vi "Tilted Logistic Square Pulse Fit Result File String.vi"(8 "error in (no error)":errorcluster, 9 "Delta Best Fit Parameters":dbl[](array[numeric]), 10 "Fit Output":T1={"best nonlinear fit"=[], "best fit parameters"=[], "R^2"=0.0, "RMSE"=0.0, "error out"={"status"=FALSE, "code"=0, "source"=""}, "Fitting Method"=enum."Least Square", "number of function calls"=0, "number of iterations"=0, "covariance"=[], "Chi 2"=0.0, "DOF"=0, "Fit Convergence Criterion"=enum."Continue", "Fitting Algorithm"=enum."Levenberg-Marquardt", "Weighted Fit"=enum."Unweighted", "Gradient"=0.0, "|Delta Chi 2|"=0.0, "|Delta Chi 2|/Chi 2"=0.0, "Max |Delta a| /|a|"=0.0, "Lambda"=-1.0, "RSS"=0.0, "AIC"=0.0, "BIC"=0.0, "Max number of function calls"=0, "Max number of iterations"=0, "IRF"={"X Array"=[], "Y Array"=[]}, "IRF Normalization Factor"=0.0, "Decay Normalization Factor"=0.0, "Number of offset fits"=0, "Weighted Chi2"=-1.0, "Unweighted Chi2"=-1.0}, 11 "ROI Descriptor":T8 {"Contours"."Type" items=["No Selection", "Point", "Line", "Rectangle", "Oval", "Polygon", "Freehand Region", "Annulus", "Unused2", "Unused3", "Broken Line", "Freehand Line", "Rotated Rectangle"]}) -> (0 "error out":errorcluster, 3 "Result String":string, 5 "Header String":string="ROI_x\tROI_y\tAL\tAL_err\tAU\tAU_err\tx0R\tx0R_err\tdxR\tdxR_err\tx0F\tx0F_err\tdxF\tdxF_err\tR^2\tRMSE\tMethod\tCalls\tIterations")   [LabVIEW 2021, in "Fits.lvlib"]
doc: "Creates Notebook output for a tilted logistic square gate fit."
uses:
  Fits.lvlib
  Non-linear Fit Output v4.ctl
  Nonlinear Fit Method.ctl
  <vilib>/Analysis/Matrix/Datatypes/RealMatrix.ctl
  Convergence Criteria.ctl
  Non-linear Fitting Algorithm.ctl
  IRF(X)PSED/Fit Weights Type v2.ctl
  Graphs/XY Graph/XY Graph Plot Data.ctl
  <vilib>/Analysis/Matrix/NI_Matrix.lvlib
  Graphs/XY Graph/XY Graph Add-Ons.lvlib
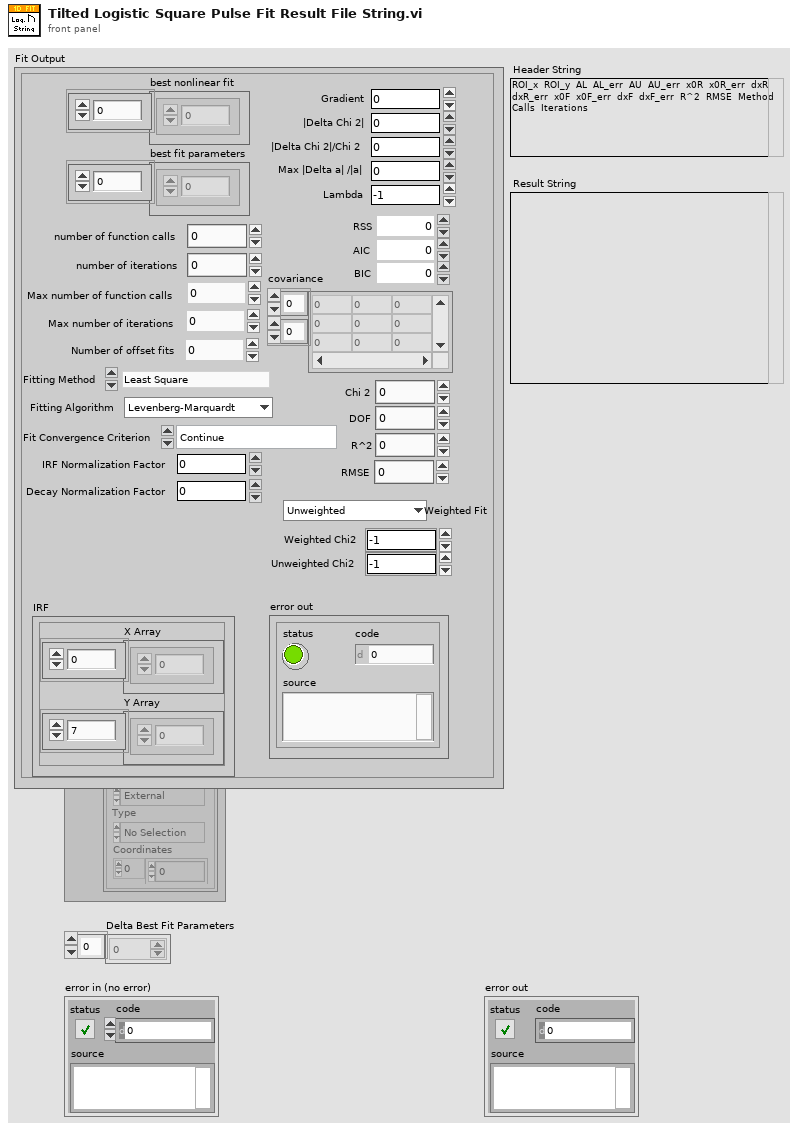
[diagram p1: front panel]
types:
  T1 = typedef "Fits.lvlib/Non-linear Fit Output v4.ctl" = cluster{"best nonlinear fit":dbl[], "best fit parameters":dbl[], "R^2":dbl, "RMSE":dbl, "error out":errorcluster, "Fitting Method":T2, "number of function calls":i32, "number of iterations":i32, "covariance":T3, "Chi 2":dbl, "DOF":i32, "Fit Convergence Criterion":T4, "Fitting Algorithm":T5, "Weighted Fit":T6, "Gradient":dbl, "|Delta Chi 2|":dbl, "|Delta Chi 2|/Chi 2":dbl, "Max |Delta a| /|a|":dbl, "Lambda":dbl, "RSS":dbl, "AIC":dbl, "BIC":dbl, "Max number of function calls":i32, "Max number of iterations":i32, "IRF":T7, "IRF Normalization Factor":dbl, "Decay Normalization Factor":dbl, "Number of offset fits":i32, "Weighted Chi2":dbl, "Unweighted Chi2":dbl}
  T2 = typedef "Fits.lvlib/Nonlinear Fit Method.ctl" = enum16{"Least Square", "Least Absolute Residual", "Bisquare", "MLE"}
  T3 = typedef "NI_Matrix.lvlib/RealMatrix.ctl" = dbl[][]
  T4 = typedef "Fits.lvlib/Convergence Criteria.ctl" = enum16{"Continue", "Tolerances Exceeded", "Max Time Exceeded", "Max Iterations Exceeded", "Max Function Evaluations Exceeded", "Scale Range Exceeded"}
  T5 = typedef "Fits.lvlib/Non-linear Fitting Algorithm.ctl" = enum16{"Levenberg-Marquardt", "Trust-Region Dogleg"}
  T6 = typedef "Fits.lvlib/Fit Weights Type v2.ctl" = enum16{"Unweighted", "1/Variance (Neyman)", "1/Variance (Pearson)", "Best of All"}
  T7 = typedef "XY Graph Add-Ons.lvlib/XY Graph Plot Data.ctl" = cluster{"X Array":dbl[], "Y Array":dbl[]}
  T8 = typedef "ROI Descriptor" = cluster{"Global Rectangle":i32[], "Contours":cluster{"ID":enum32{"External", "Internal"}, "Type":u32, "Coordinates":i32[]}[]}
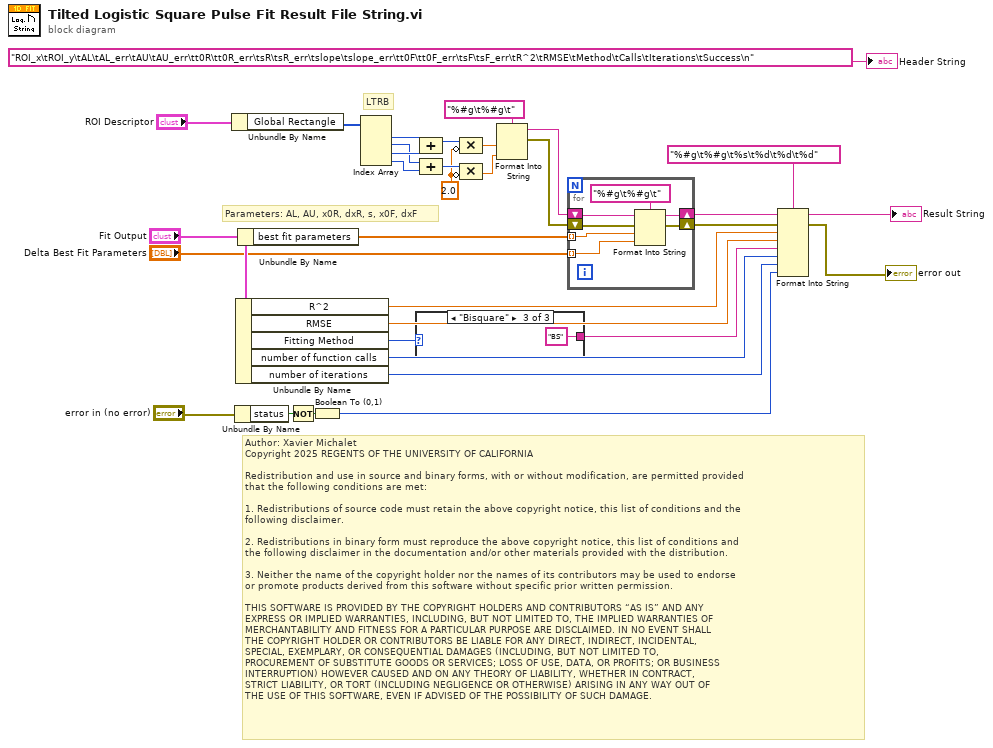
[diagram p0: block diagram]
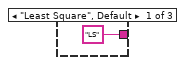
[diagram p2: hidden frame]
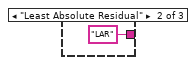
[diagram p3: hidden frame]
diagram:
  w7 = 2.0 ("value")
  # "Author: Xavier Michalet\nCopyright 2025 REGENTS OF THE UNIVERSITY OF CALIFORNIA\n\nRedistribution and use in source and binary forms, with or without modification, are permitted provided\nthat the following conditions are met:\n\n1. Redistributions of source code must retain the above copyright notice, this list of conditions and the\nfollowing disclaimer.\n\n2. Redistributions in binary form must reproduce the above copyright notice, this list of conditions and\nthe following disclaimer in the documentation and/or other materials provided with the distribution.\n\n3. Neither the name of the copyright holder nor the names of its contributors may be used to endorse \nor promote products derived from this software without specific prior written permission.\n\nTHIS SOFTWARE IS PROVIDED BY THE COPYRIGHT HOLDERS AND CONTRIBUTORS “AS IS” AND ANY \nEXPRESS OR IMPLIED WARRANTIES, INCLUDING, BUT NOT LIMITED TO, THE IMPLIED WARRANTIES OF\nMERCHANTABILITY AND FITNESS FOR A PARTICULAR PURPOSE ARE DISCLAIMED. IN NO EVENT SHALL\nTHE COPYRIGHT HOLDER OR CONTRIBUTORS BE LIABLE FOR ANY DIRECT, INDIRECT, INCIDENTAL, \nSPECIAL, EXEMPLARY, OR CONSEQUENTIAL DAMAGES (INCLUDING, BUT NOT LIMITED TO, \nPROCUREMENT OF SUBSTITUTE GOODS OR SERVICES; LOSS OF USE, DATA, OR PROFITS; OR BUSINESS\nINTERRUPTION) HOWEVER CAUSED AND ON ANY THEORY OF LIABILITY, WHETHER IN CONTRACT, \nSTRICT LIABILITY, OR TORT (INCLUDING NEGLIGENCE OR OTHERWISE) ARISING IN ANY WAY OUT OF\nTHE USE OF THIS SOFTWARE, EVEN IF ADVISED OF THE POSSIBILITY OF SUCH DAMAGE."
  # "LTRB"
  # "Parameters: AL, AU, x0R, dxR, s, x0F, dxF"
  n1 = Unbundle By Name("ROI Descriptor") -> ("Global Rectangle"=w15:i32[])
  n2 = Unbundle By Name("error in (no error)") -> ("status"=w4:bool)
  n3 = Unbundle By Name("Fit Output") -> ("R^2"=w21:dbl, "RMSE"=w20:dbl, "Fitting Method"=w19:T2, "number of function calls"=w17:i32, "number of iterations"=w16:i32)
  n4 = Unbundle By Name("Fit Output") -> ("best fit parameters"=w27:dbl[])
  n5 = Not(x=w4) -> (.not. x?=w3:bool)
  n6 = Boolean To (0,1)(Boolean=w3) -> (0, 1=w1:i16)
  n7 = Index Array(array=w15) -> (element #1=w14:i32, element #2=w11:i32, element #3=w13:i32, element #4=w12:i32)  [unwired: 4 in]
  n8 = case shown="\"Bisquare\"" w19 {
    tunnel: ["LS" ("input 3") "LAR" ("input 3") "BS" ("input 3")] -> w18
    frame "Least Square", Default {
    }
    frame "Least Absolute Residual" {
    }
    frame "Bisquare" {
    }
  }
  n9 = Compound Arithmetic op=ADD(w14, w13) -> (w9:i32)
  n10 = Compound Arithmetic op=ADD(w11, w12) -> (w8:i32)
  n11 = Compound Arithmetic op=MULTIPLY(w9, invert w7) -> (w6:dbl)
  n12 = Compound Arithmetic op=MULTIPLY(w8, invert w7) -> (w5:dbl)
  n13 = Format Into String(format string="%#g\t%#g\t", w6, w5) -> (resulting string=w25:string, error out=w26:errorcluster)  [unwired: 2 in]
  n14 = for {
    tunnel: w27 -> [w42] mode=indexing
    tunnel: "Delta Best Fit Parameters" -> [w41] mode=indexing
    shift-right: [w39] -> w24
    shift-left: w25 -> [w40]
    shift-right: [w38] -> w23
    shift-left: w26 -> [w37]
    n15 = Format Into String(format string="%#g\t%#g\t", initial string=w40, error in=w37, w42, w41) -> (resulting string=w39:string, error out=w38:errorcluster)
  }
  n16 = Format Into String(format string="%#g\t%#g\t%s\t%d\t%d\t%d", initial string=w24, error in=w23, w21, w20, w18, w17, w16, w1) -> (resulting string=→"Result String":string, error out=→"error out":errorcluster)
  "Header String" <- "ROI_x\tROI_y\tAL\tAL_err\tAU\tAU_err\tt0R\tt0R_err\tsR\tsR_err\tslope\tslope_err\tt0F\tt0F_err\tsF\tsF_err\tR^2\tRMSE\tMethod\tCalls\tIterations\tSuccess\n" ("format string")
